vi "dfd_Group Delay_Interpolate Band Grid Points.vi"(2 "nominal df":dbl, 3 "f":dbl[](array[numeric])) -> (0 "delta f":dbl[](array[numeric]), 1 "interpolated f":dbl[](array[numeric]))   [LabVIEW 2017, in "NI_DigFilter_Design.lvlib"]
uses:
  <vilib>/addons/Digital Filter Design/NI_DigFilter_Design.lvlib
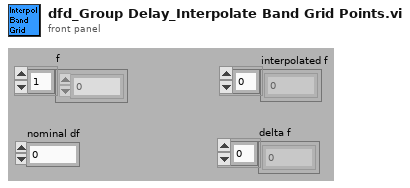
[diagram p1: front panel]
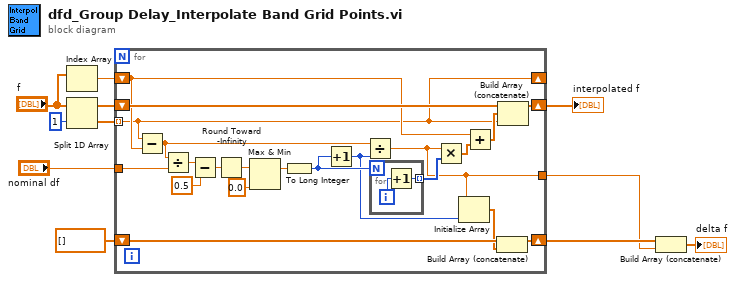
[diagram p0: block diagram]
diagram:
  n1 = Index Array(array="f") -> (element=w7:dbl)  [unwired: 1 in]
  n2 = Split 1D Array(array="f", index=1) -> (first subarray=w10:dbl[], second subarray=w9:dbl[])
  n3 = for {
    shift-right: [w31] -> w6
    shift-left: w10 -> [w32]
    tunnel: w9 -> [w24] mode=indexing
    shift-right: [w24] -> _
    shift-left: w7 -> [w28]
    tunnel: "nominal df" -> [w21]
    shift-right: [w27] -> w3
    shift-left: dbl[] [] -> [w25]
    tunnel: [w23] -> w1
    n4 = Subtract(x=w24, y=w28) -> (x-y=w20:dbl)
    n5 = Divide(x=w20, y=w21) -> (x/y=w18:dbl)
    n6 = Subtract(x=w18, y=0.5) -> (x-y=w19:dbl)
    n7 = Round Toward -Infinity(1:w19) -> (0:w16:dbl)
    n8 = Max & Min(x=w16, y=0.0) -> (max(x,y)=w14:dbl)  [unwired: 1 out]
    n9 = To Long Integer(number=w14) -> (32bit integer=w13:i32)
    n10 = Increment(x=w13) -> (x+1=w12:i32)
    n11 = Divide(x=w20, y=w12) -> (x/y=w23:dbl)
    n12 = for {
      N: w13 -> [_]
      tunnel: [w33] -> w30 mode=indexing
      i -> [w34]
      n13 = Increment(x=w34) -> (x+1=w33:i32)
    }
    n14 = Multiply(x=w23, y=w30) -> (x*y=w29:dbl[])
    n15 = Initialize Array(w23, w12) -> (w22:dbl[])
    n16 = Add(x=w28, y=w29) -> (x+y=w26:dbl[])
    n17 = Build Array (concatenate)(w25, w22) -> (w27:dbl[])
    n18 = Build Array (concatenate)(w32, w26, w24) -> (w31:dbl[])
  }
  "interpolated f" <- w6
  n19 = Build Array (concatenate)(w3, w1) -> (→"delta f":dbl[])
